vi "CreateDataFolders.vi"(8 "Location In":T1=enum."WCM Main", 10 "Create Data Folder":bool, 11 "Data Drive":string) -> ()   [LabVIEW 2022 SP3]
uses:
  ScanningControl/-ScanSystem/Controls/location.ctl
  ScanningControl/Motion Controllers/-MotionRoutines/MotionGlobals.vi
  Patient Routines/PatientGlobals.vi
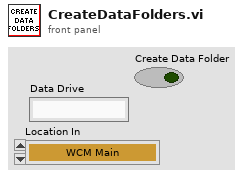
[diagram p1: front panel]
types:
  T1 = typedef "location.ctl" = enum16{"Automatic", "WCM Main", "Hawaii", "Columbia MM3000", "Columbia  NI System", "NYU", "RRI 2", "UHI Allen", "CUMC RT", "Chiba", "Stony Brook", "WCM Microscopy", "WCM Aeoretch", "WCM Optics Lab", "WCM Main 2Axis", "WCM Rotation", "WCM SAM SMAC", "SERI GP"}
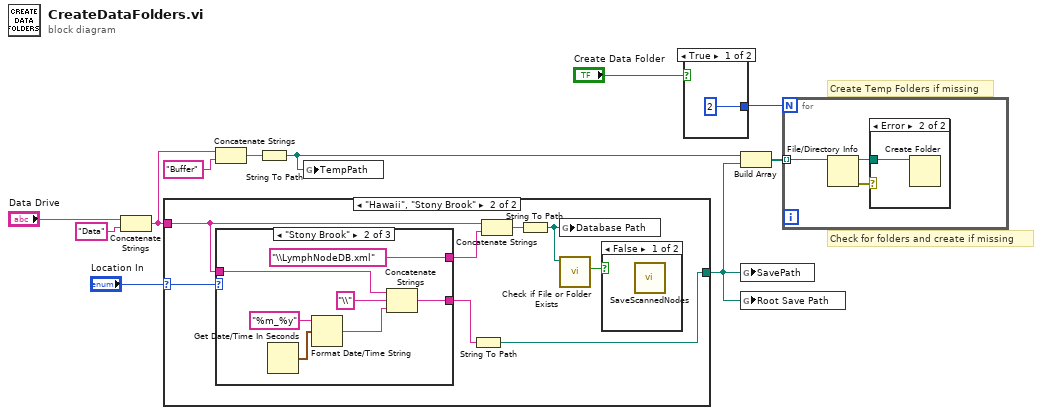
[diagram p0: block diagram]
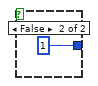
[diagram p2: hidden frame]
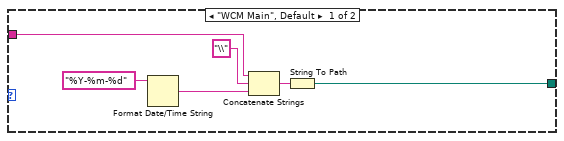
[diagram p3: hidden frame]
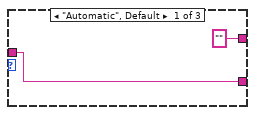
[diagram p5: hidden frame]
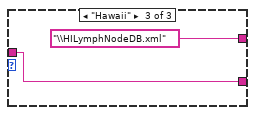
[diagram p6: hidden frame]
diagram:
  # "Create Temp Folders if missing"
  # "Check for folders and create if missing"
  n1 = Concatenate Strings("Data Drive", "Data" ("name or relative path")) -> (w9:string)
  n2 = case shown="\"Hawaii\", \"Stony Brook\"" "Location In" {
    selector: "Location In" -> [_ w22]
    tunnel: [w17 w25] -> w4
    tunnel: w9 -> [w16 w19]
    frame "WCM Main", Default {
      n3 = Format Date/Time String(time format string (%c)="%Y-%m-%d") -> (date/time string=w14:string)  [unwired: 2 in]
      n4 = Concatenate Strings(w16, "\\" ("string"), w14) -> (w15:string)
      n5 = String To Path(string=w15) -> (path=w17:path)
    }
    frame "Hawaii", "Stony Brook" {
      n6 = case shown="\"Stony Brook\"" w22 {
        tunnel: ["" ("string") "\\LymphNodeDB.xml" ("string") "\\HILymphNodeDB.xml" ("string")] -> w24
        tunnel: w19 -> [w26 w31 w35]
        tunnel: [w26 w28 w35] -> w18
        frame "Automatic", Default {
        }
        frame "Stony Brook" {
          n7 = Get Date/Time In Seconds() -> (seconds since 1Jan1904=w32:timestamp)
          n8 = Format Date/Time String(time format string (%c)="%m_%y", seconds (now)=w32) -> (date/time string=w29:string)  [unwired: 1 in]
          n9 = Concatenate Strings(w31, "\\" ("string"), w29) -> (w28:string)
        }
        frame "Hawaii" {
        }
      }
      n10 = String To Path(string=w18) -> (path=w25:path)
      n11 = Concatenate Strings(w19, w24) -> (w23:string)
      n12 = String To Path(string=w23) -> (path=w20:path)
      n13 = global write "PatientGlobals.vi" "Database Path"(w20) -> ()
      n14 = call <vilib>:"Check if File or Folder Exists.vi"("path"=w20) -> ("file or folder exists?"=w21:bool)  [unwired: 8 in, 2 out]
      n15 = case shown="False" w21 {
        frame False {
          n16 = call "SaveScannedNodes.vi"() -> ()  [unwired: 12 in]
        }
        frame True {
        }
      }
    }
  }
  n17 = Concatenate Strings(w9, "Buffer" ("name or relative path")) -> (w7:string)
  n18 = String To Path(string=w7) -> (path=w2:path)
  n19 = global write "MotionGlobals.vi" "TempPath"(w2) -> ()
  n20 = case shown="True" "Create Data Folder" {
    tunnel: [2 1] -> w3
    frame True {
    }
    frame False {
    }
  }
  n21 = Build Array(w2, w4) -> (w6:path[])
  n22 = global write "MotionGlobals.vi" "SavePath"(w4) -> ()
  n23 = global write "MotionGlobals.vi" "Root Save Path"(w4) -> ()
  n24 = for {
    N: w3 -> [_]
    tunnel: w6 -> [w39] mode=indexing
    n25 = File/Directory Info(path=w39) -> (path out=w40:path, error out=w41:errorcluster)  [unwired: 1 in, 5 out]
    n26 = case shown="Error" w41 {
      tunnel: w40 -> [_ w42]
      frame No Error {
      }
      frame Error {
        n27 = Create Folder(path (use dialog)=w42) -> ()  [unwired: 1 in, 4 out]
      }
    }
  }
